vi "Winkel Task Beenden.vi"(8 "error IO":errorcluster, 10 "Task In":T1) -> (0 "error out":errorcluster)   [LabVIEW 2014]
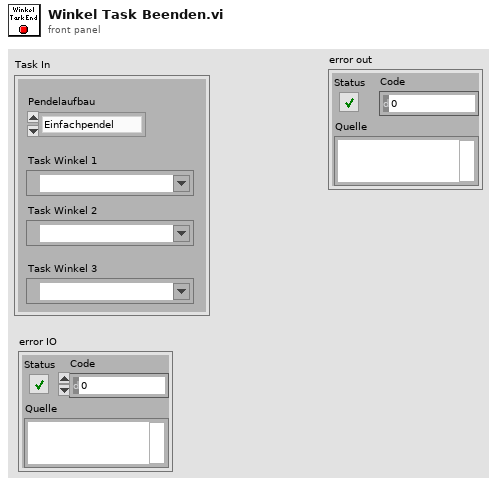
[diagram p1: front panel]
types:
  T1 = cluster{"Pendelaufbau":enum16{"Einfachpendel", "Doppelpendel", "Dreifachpendel"}, "task/channels in":refnum<k21>, "task/channels in 2":refnum<k21>, "task/channels in 3":refnum<k21>}
  T2 = enum16{"Einfachpendel", "Doppelpendel", "Dreifachpendel"}
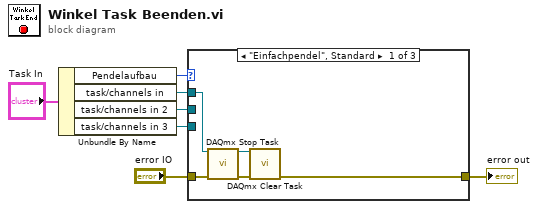
[diagram p0: block diagram]
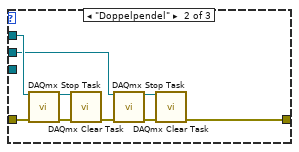
[diagram p2: hidden frame]
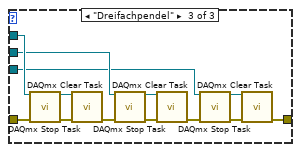
[diagram p3: hidden frame]
diagram:
  n1 = Unbundle By Name("Task In") -> ("Pendelaufbau"=w1:T2, "task/channels in"=w5:refnum<k21>, "task/channels in 2"=w4:refnum<k21>, "task/channels in 3"=w3:refnum<k21>)
  n2 = case shown="\"Einfachpendel\", Standard" w1 {
    tunnel: "error IO" -> [w9 w15 w25]
    tunnel: [w12 w17 w28] -> w2
    tunnel: w5 -> [w8 w14 w24]
    tunnel: w4 -> [_ w13 w23]
    tunnel: w3 -> [_ _ w22]
    frame "Einfachpendel", Default {
      n3 = call <vilib>:"DAQmx Stop Task.vi"("task/channels in"=w8, "error in"=w9) -> ("task out"=w11:refnum<k21>, "error out"=w10:errorcluster)  [unwired: 12 in]
      n4 = call <vilib>:"DAQmx Clear Task.vi"("task in"=w11, "error in"=w10) -> ("error out"=w12:errorcluster)  [unwired: 13 in]
    }
    frame "Doppelpendel" {
      n5 = call <vilib>:"DAQmx Stop Task.vi"("task/channels in"=w14, "error in"=w15) -> ("task out"=w21:refnum<k21>, "error out"=w20:errorcluster)  [unwired: 12 in]
      n6 = call <vilib>:"DAQmx Clear Task.vi"("task in"=w21, "error in"=w20) -> ("error out"=w16:errorcluster)  [unwired: 13 in]
      n7 = call <vilib>:"DAQmx Stop Task.vi"("task/channels in"=w13, "error in"=w16) -> ("task out"=w19:refnum<k21>, "error out"=w18:errorcluster)  [unwired: 12 in]
      n8 = call <vilib>:"DAQmx Clear Task.vi"("task in"=w19, "error in"=w18) -> ("error out"=w17:errorcluster)  [unwired: 13 in]
    }
    frame "Dreifachpendel" {
      n9 = call <vilib>:"DAQmx Stop Task.vi"("task/channels in"=w24, "error in"=w25) -> ("task out"=w34:refnum<k21>, "error out"=w33:errorcluster)  [unwired: 12 in]
      n10 = call <vilib>:"DAQmx Clear Task.vi"("task in"=w34, "error in"=w33) -> ("error out"=w27:errorcluster)  [unwired: 13 in]
      n11 = call <vilib>:"DAQmx Stop Task.vi"("task/channels in"=w23, "error in"=w27) -> ("task out"=w32:refnum<k21>, "error out"=w31:errorcluster)  [unwired: 12 in]
      n12 = call <vilib>:"DAQmx Clear Task.vi"("task in"=w32, "error in"=w31) -> ("error out"=w26:errorcluster)  [unwired: 13 in]
      n13 = call <vilib>:"DAQmx Stop Task.vi"("task/channels in"=w22, "error in"=w26) -> ("task out"=w30:refnum<k21>, "error out"=w29:errorcluster)  [unwired: 12 in]
      n14 = call <vilib>:"DAQmx Clear Task.vi"("task in"=w30, "error in"=w29) -> ("error out"=w28:errorcluster)  [unwired: 13 in]
    }
  }
  "error out" <- w2
